vi "Handle Panel Close.vi"(8 "error in (no error)":errorcluster, 11 "OneButtonDialogBox In":refnum<class "OneButtonDialogBox.lvclass">) -> (0 "error out":errorcluster, 3 "OneButtonDialogBox Out":refnum<class "OneButtonDialogBox.lvclass">)   [LabVIEW 2015, in "OneButtonDialogBox.lvlib" / "OneButtonDialogBox.lvclass"]
uses:
  OneButtonDialogBox.lvclass
  <vilib>/ActorFramework/Actor/Actor.lvclass/Actor.ctl
  <vilib>/ActorFramework/Message Enqueuer/Message Enqueuer.lvclass/Message Enqueuer.ctl
  OneButtonDialogBox.lvclass/OneButtonDialogBox.ctl
  <vilib>/ActorFramework/Message Enqueuer/Init from Existing Queue.vi
  <vilib>/ActorFramework/Message Enqueuer/Enqueue.vi
  <vilib>/ActorFramework/Message Priority Queue/Priority Enqueue.vi
  <vilib>/ActorFramework/Message Enqueuer/Message Enqueuer.lvclass
  <vilib>/ActorFramework/Stop Msg/Stop Msg.lvclass
  IDialogBox/IDialogBox Abstract Messages/Abstract Dialog Return Msg/Abstract Dialog Return Msg.lvclass
  <vilib>/ActorFramework/Actor/Actor.lvclass
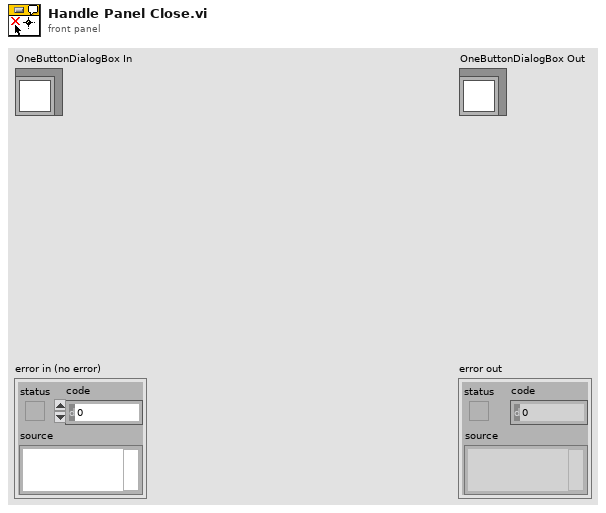
[diagram p1: front panel]
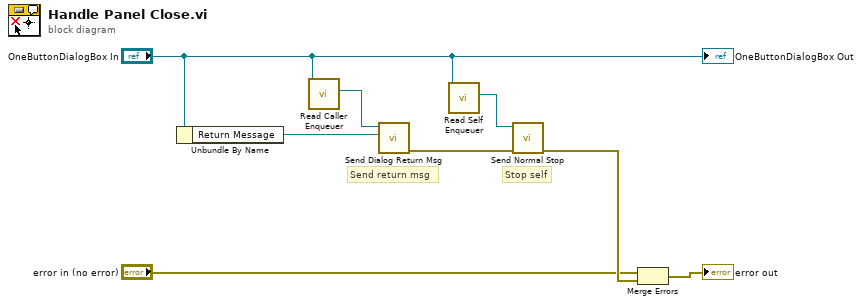
[diagram p0: block diagram]
diagram:
  # "Stop self"
  # "Send return msg"
  n1 = Unbundle By Name("OneButtonDialogBox In") -> ("Return Message"=w8:refnum<class "Abstract Dialog Return Msg.lvclass">)
  n2 = call <vilib>:"Read Caller Enqueuer.vi"("Actor"="OneButtonDialogBox In") -> ("Caller Enqueuer"=w7:refnum<class "Message Enqueuer.lvclass">)  [unwired: 10 in]
  n3 = call "Send Dialog Return Msg.vi"("Dialog Return Msg"=w8, "Message Enqueuer in"=w7) -> ("error out"=w5:errorcluster)  [unwired: 9 in]
  n4 = call <vilib>:"Read Self Enqueuer.vi"("Actor"="OneButtonDialogBox In") -> ("Self Enqueuer"=w6:refnum<class "Message Enqueuer.lvclass">)  [unwired: 10 in]
  n5 = call <vilib>:"Send Normal Stop.vi"("error in (no error)"=w5, "Message Enqueuer"=w6) -> ("error out"=w4:errorcluster)  [unwired: 9 in]
  n6 = Merge Errors("error in (no error)", w4) -> (→"error out":errorcluster)
  "OneButtonDialogBox Out" <- "OneButtonDialogBox In"
